vi "XY Plot - Y Scale - Marker Width--Const.vi"() -> (3 "Y Scale.Marker.Size:Width":u32)   [LabVIEW 2017, in "DTacq Plot Display Library.lvlib"]
uses:
  DTacq Plot Display Library.lvlib
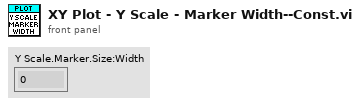
[diagram p1: front panel]
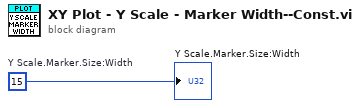
[diagram p0: block diagram]
diagram:
  w1 = u32 15  # Y Scale.Marker.Size:Width
  "Y Scale.Marker.Size:Width" <- w1
